vi "Get Pressure.vi"(8 "error in (no error)":errorcluster, 11 "GaugeController in":refnum<class "GaugeController.lvclass">) -> (0 "error out":errorcluster, 2 "Pressure":dbl[](array[numeric]), 3 "GaugeController out":refnum<class "GaugeController.lvclass">)   [LabVIEW 2016, in "Hardware.lvlib" / "GaugeController.lvlib" / "GaugeController.lvclass"]
uses:
  <userlib>/Common Components/Hardware/GaugeController/GaugeController/GaugeController.lvclass
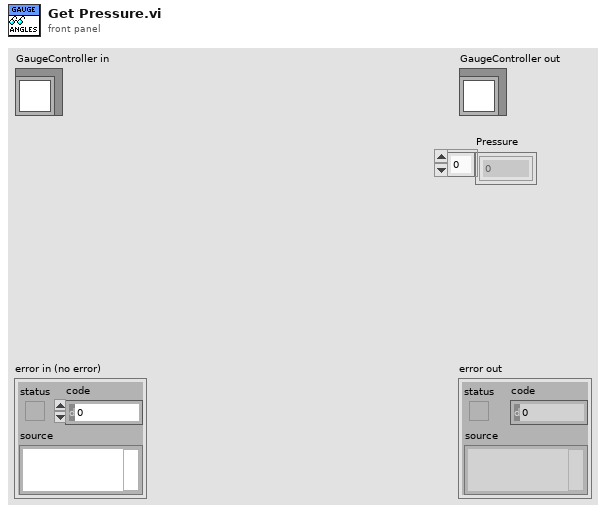
[diagram p1: front panel]
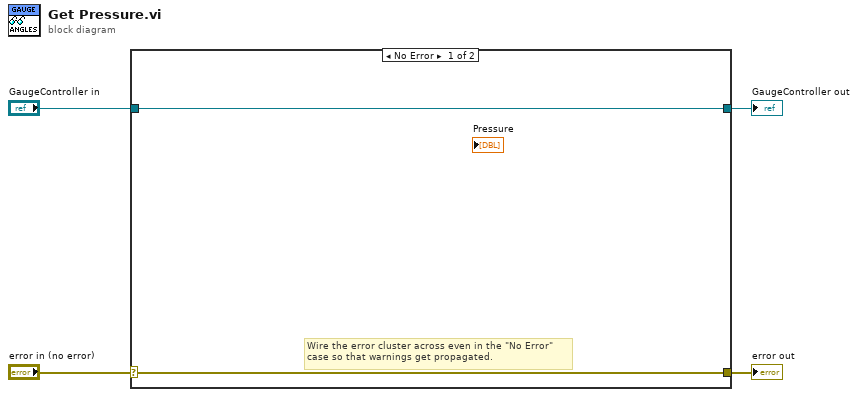
[diagram p0: block diagram]
diagram:
  n1 = case shown="No Error" "error in (no error)" {
    selector: "error in (no error)" -> [w5 w8]
    tunnel: [w5 w8] -> w3
    tunnel: [w6 w7] -> w1
    tunnel: "GaugeController in" -> [w6 w7]
    frame No Error {
      # "Wire the error cluster across even in the \"No Error\"\ncase so that warnings get propagated."
    }
    frame Error {
    }
  }
  "error out" <- w3
  "GaugeController out" <- w1
